vi "RunO3Lamp.vi"(7 "LVWSR":refnum<class "Web Request.lvclass">, 11 "Run":u8) -> ()   [LabVIEW 2014]
uses:
  Calibration/O3 Frequency Train Actor/Messages/Run/Change O3 Lamp Run MSG.lvclass
  Controller/Controller.lvclass
  Controller/Controls/Enqueuer Enum.ctl
  <vilib>/wsapi/Web Request.lvclass
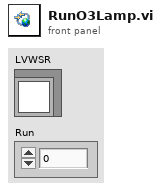
[diagram p1: front panel]
types:
  T1 = typedef "Controller.lvlib/Controller.lvclass/Enqueuer Enum.ctl" = enum8{"PAS", "CRDS", "File", "O3Lamp"}
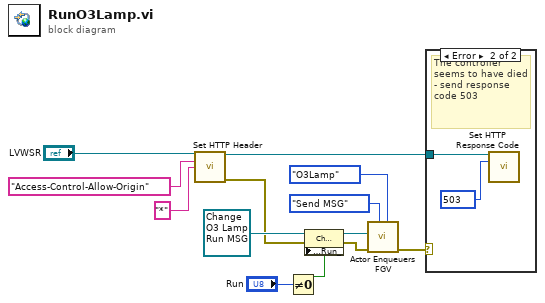
[diagram p0: block diagram]
diagram:
  n1 = call <vilib>:"Set HTTP Header.vi"("LabVIEW Web Service Request"="LVWSR", "header"="Access-Control-Allow-Origin", "header value"="*") -> ("LabVIEW Web Service Request out"=w8:refnum<class "Web Request.lvclass">, "error out"=w2:errorcluster)  [unwired: 11 in]
  n2 = Not Equal To 0?(x="Run") -> (x != 0?=w5:bool)
  n3 = property class="Change O3 Lamp Run MSG.lvclass"(reference=refnum<class "Change O3 Lamp Run MSG.lvclass"> refnum ("Calibration.lvlib:Change O3 Lamp Run"), error in=w2, "Accessors:Run_"=w5) -> (reference out=w4:refnum<class "Change O3 Lamp Run MSG.lvclass">, error out=w1:errorcluster)
  n4 = call "Actor Enqueuers FGV.vi"("Enqueuer"=Enqueuer_Enum."O3Lamp", "State"=enum16{"Store", "Send MSG"}."Send MSG", "error in"=w1, "MSG"=w4) -> ("error out"=w3:errorcluster)  [unwired: 7 in]
  n5 = case shown="Error" w3 {
    tunnel: w8 -> [_ w14]
    frame No Error {
    }
    frame Error {
      w15 = 503 items=["100"=100, "101"=101, "200"=200, "201"=201, "202"=202, "203"=203, "204"=204, "205"=205, "206"=206, "300"=300, "301"=301, "302"=302, "303"=303, "304"=304, "305"=305, "306"=306, "307"=307, "400"=400, "401"=401, "402"=402, "403"=403, "404"=404, "405"=405, "406"=406, "407"=407, "408"=408, "409"=409, "410"=410, "411"=411, "412"=412, "413"=413, "414"=414, "415"=415, "416"=416, "417"=417, "500"=500, "501"=501, "502"=502, "503"=503, "504"=504, "505"=505] ("response code (200)")
      # "The controller seems to have died - send response code 503"
      n6 = call <vilib>:"Set HTTP Response Code.vi"("LabVIEW Web Service Request"=w14, "response code (200)"=w15) -> ()  [unwired: 12 in, 2 out]
    }
  }
